vi "h5_write_2d_double_array.vi"(0 "h5 dir ref":i32, 1 "dataset name":string, 5 "array":dbl[][](array[numeric]), 7 "units (au)":string="au", 11 "error in (no error)":errorcluster, 12 "dim1 (index)":string="index", 13 "dim2 (index)":string="index") -> (4 "h5 obj ref":i32, 15 "error out":errorcluster)   [LabVIEW 2015]
uses:
  <userlib>/_OpenG.lib/string/string.llb/To Camel Case (String)__ogtk.vi
  <vilib>/addons/h5labview2/base/lib_path.vi
  <vilib>/addons/h5labview2/base/H5Equery.vi
  <vilib>/addons/h5labview2/dataset/H5Dwrite.llb/H5Dwrite.xnode
  <vilib>/addons/h5labview2/attrib/H5Awrite.llb/H5Awrite.xnode
panel:
  # "Dim1 is the most recently added dimention. In general, DimN is changing faster the larger the N - C convention. - MK"
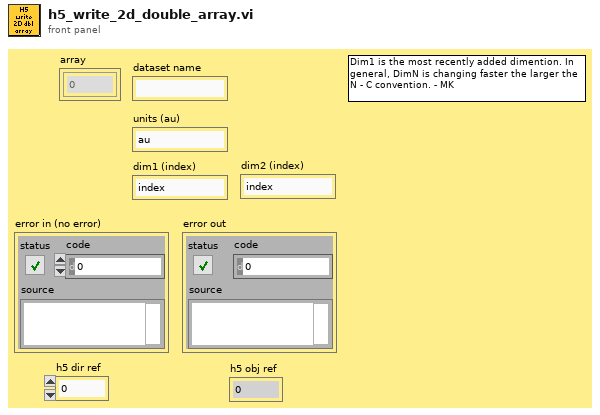
[diagram p1: front panel]
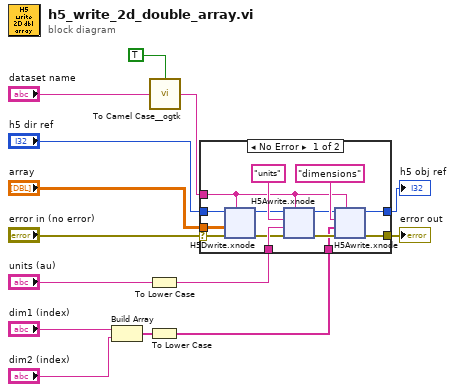
[diagram p0: block diagram]
diagram:
  n1 = Build Array("dim1 (index)", "dim2 (index)") -> (w5:string[])
  n2 = To Lower Case(string="units (au)") -> (all lower case string=w3:string)
  n3 = To Lower Case(string=w5) -> (all lower case string=w4:string[])
  n4 = call-poly <userlib>:"To Camel Case__ogtk.vi"("string"="dataset name", "no change if no spaces? (F=No)"=TRUE) -> ("CamelCase string"=w2:string)
  n5 = case shown="No Error" "error in (no error)" {
    selector: "error in (no error)" -> [w16 w87]
    tunnel: "h5 dir ref" -> [w28 w86]
    tunnel: w3 -> [w26 _]
    tunnel: "array" -> [w24 _]
    tunnel: w2 -> [w19 _]
    tunnel: [w18 w87] -> w12
    tunnel: [w17 w86] -> w11
    tunnel: w4 -> [w15 _]
    frame No Error {
      n6 = xnode "H5Dwrite.xnode"("dataset name"=w19, "error in (no error)"=w16, "data"=w24, "ref in"=w28) -> ("error out"=w23:errorcluster, "ref out"=w21:i32)  [unwired: 3 in, 1 out]
      n7 = xnode "H5Awrite.xnode"("object name"=w19, "error in (no error)"=w23, "data"=w26, "attrib name"="units", "ref in"=w21) -> ("error out"=w22:errorcluster, "ref out"=w20:i32)  [unwired: 2 in, 1 out]
      n8 = xnode "H5Awrite.xnode"("object name"=w19, "error in (no error)"=w22, "data"=w15, "attrib name"="dimensions", "ref in"=w20) -> ("error out"=w18:errorcluster, "ref out"=w17:i32)  [unwired: 2 in, 1 out]
    }
    frame Error {
    }
  }
  "error out" <- w12
  "h5 obj ref" <- w11
